vi "DT_Triangle Manager_Init Edge.vi"(8 "right point":i32, 9 "left point":i32, 10 "next triangle in":i32, 11 "Triangles In":i32[][](array[numeric])) -> (2 "next triangle out":i32, 3 "Triangles Out":i32[][](array[numeric]))   [LabVIEW 2020, in "NI_AAL_Geometry.lvlib"]
uses:
  <vilib>/Analysis/NI_AAL_Geometry.lvlib
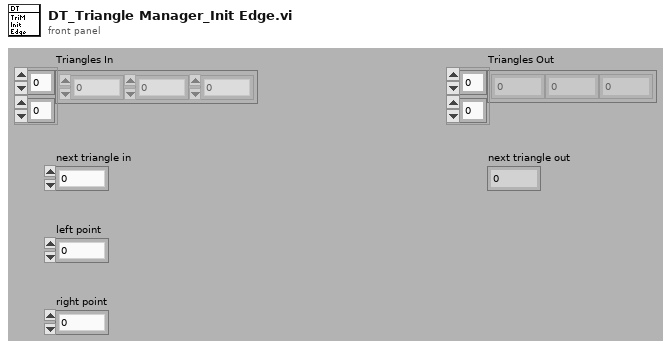
[diagram p1: front panel]
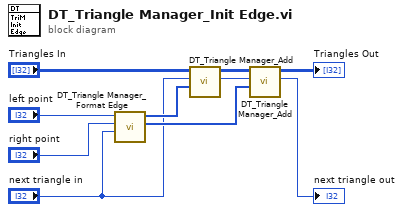
[diagram p0: block diagram]
diagram:
  n1 = call <vilib>:"DT_Triangle Manager_Format Edge.vi"("start triangle"="next triangle in", "point 2"="right point", "point 1"="left point") -> ("Second Triangle"=w2:i32[], "First Triangle"=w3:i32[])  [unwired: 7 out]
  n2 = call <vilib>:"DT_Triangle Manager_Add.vi"("Triangle"=w3, "next triangle in"="next triangle in", "Triangles In"="Triangles In") -> ("next triangle out"=w6:i32, "Triangles Out"=w7:i32[][])  [unwired: 7 out]
  n3 = call <vilib>:"DT_Triangle Manager_Add.vi"("Triangle"=w2, "next triangle in"=w6, "Triangles In"=w7) -> ("next triangle out"=→"next triangle out":i32, "Triangles Out"=→"Triangles Out":i32[][])  [unwired: 7 out]
